vi "IviChannelsToProperty.vi"(8 "error in (no error)":errorcluster, 11 "IVI_Class.lvclass":refnum<class "IVI_Class.lvclass">) -> (0 "error out":errorcluster, 3 "IVI_Class.lvclass":refnum<class "IVI_Class.lvclass">)   [LabVIEW 2014, in "ScopePlugins.lvlib" / "IVI_Class.lvclass"]
doc: "Reads IVI Scope Acquisition properties and writes them into the Scope class Acquisition Properties"
uses:
  IVI_Class.lvclass
  ScopePluginBaseClass/ScopePluginsBase.lvclass/ScopePluginsBase.ctl
  ScopePluginBaseClass/Accessors/Write Channels.vi
  ScopePluginBaseClass/Accessors/Read Handle.vi
  ScopePluginBaseClass/Accessors/Read Connected.vi
  ScopePluginBaseClass/Accessors/Read Channels.vi
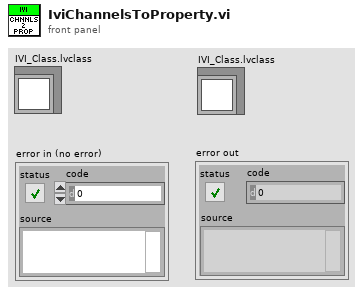
[diagram p1: front panel]
types:
  T1 = typedef "ScopePlugins.lvlib/Channels.ctl" = cluster{"Count":i32, "ChannelArray":T2[]}
  T2 = typedef "ScopePlugins.lvlib/Channel.ctl" = cluster{"Enabled":bool, "Name":string, "InputImpedance":dbl, "InputFreqMax":dbl, "ProbeAttn":dbl, "Coupling":enum16{"AC", "DC", "GND"}, "Offset":dbl, "Range":dbl}
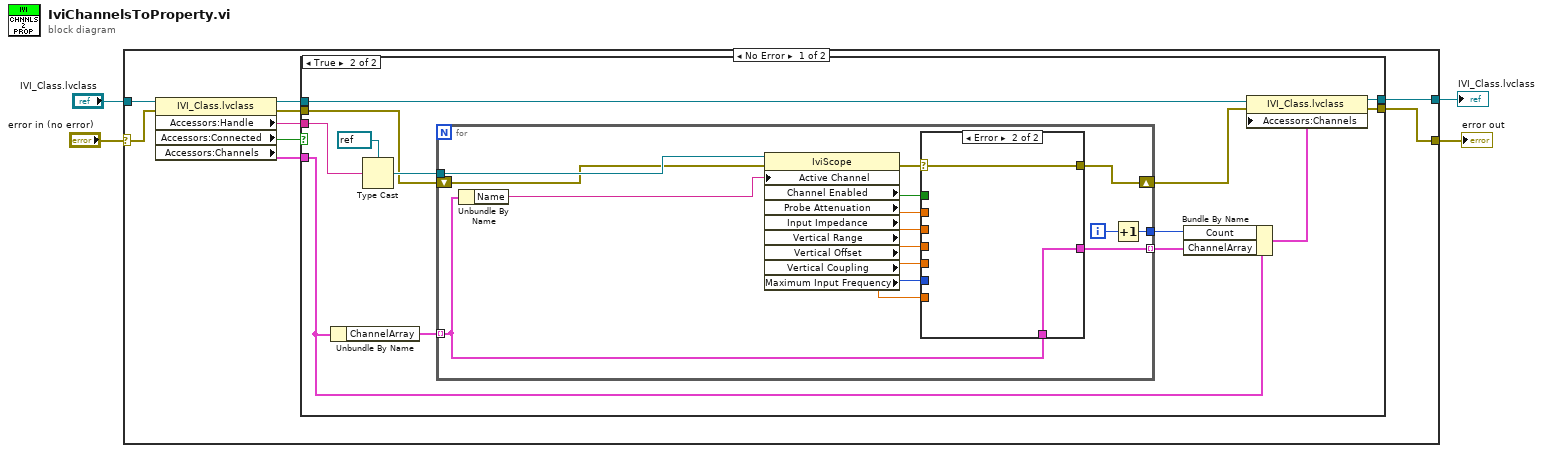
[diagram p0: block diagram]
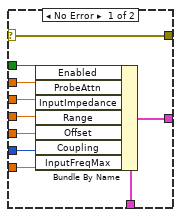
[diagram p3: hidden frame]
diagram:
  n1 = case shown="No Error" "error in (no error)" {
    selector: "error in (no error)" -> [w9 w57]
    tunnel: "IVI_Class.lvclass" -> [w13 w58]
    tunnel: [w10 w58] -> w3
    tunnel: [w7 w57] -> w1
    frame No Error {
      n2 = property class="IVI_Class.lvclass"(reference=w13, error in=w9) -> (reference out=w11:refnum<class "IVI_Class.lvclass">, error out=w8:errorcluster, "Accessors:Handle"=w12:string, "Accessors:Connected"=w6:bool, "Accessors:Channels"=w5:T1)
      n3 = case shown="True" w6 {
        tunnel: w12 -> [_ w27]
        tunnel: w11 -> [w15 w20]
        tunnel: [w15 w25] -> w10
        tunnel: w8 -> [w14 w24]
        tunnel: [w14 w22] -> w7
        tunnel: w5 -> [_ w19]
        frame False {
        }
        frame True {
          n4 = Unbundle By Name(w19) -> ("ChannelArray"=w21:T2[])
          n5 = Type Cast(type=refnum<k15> refnum ("reference out"), x=w27) -> (*(type *) &x=w26:refnum<k15>)
          n6 = for {
            tunnel: w26 -> [w39]
            shift-right: [w40] -> w23
            shift-left: w24 -> [w38]
            tunnel: w21 -> [w44] mode=indexing
            tunnel: [w43] -> w18 mode=indexing
            tunnel: [w29] -> w16
            i -> [w42]
            n7 = Unbundle By Name(w44) -> ("Name"=w37:string)
            n8 = property class="IviScope"(reference=w39, error in=w38, "Active Channel"=w37) -> (error out=w41:errorcluster, "Channel Enabled"=w36:bool, "Probe Attenuation"=w35:dbl, "Input Impedance"=w34:dbl, "Vertical Range"=w33:dbl, "Vertical Offset"=w32:dbl, "Vertical Coupling"=w31:i32, "Maximum Input Frequency"=w30:dbl)  [unwired: 1 out]
            n9 = case shown="Error" w41 {
              selector: w41 -> [w46 w56]
              tunnel: w44 -> [w54 w55]
              tunnel: [w53 w55] -> w43
              tunnel: w35 -> [w52 _]
              tunnel: w33 -> [w51 _]
              tunnel: w32 -> [w50 _]
              tunnel: w31 -> [w49 _]
              tunnel: w30 -> [w48 _]
              tunnel: w34 -> [w47 _]
              tunnel: [w46 w56] -> w40
              tunnel: w36 -> [w45 _]
              frame No Error {
                n10 = Bundle By Name(cluster=w54, "Enabled"=w45, "ProbeAttn"=w52, "InputImpedance"=w47, "Range"=w51, "Offset"=w50, "Coupling"=w49, "InputFreqMax"=w48) -> (w53:T2)
              }
              frame Error {
              }
            }
            n11 = Increment(x=w42) -> (x+1=w29:i32)
          }
          n12 = Bundle By Name(cluster=w19, "Count"=w16, "ChannelArray"=w18) -> (w17:T1)
          n13 = property class="IVI_Class.lvclass"(reference=w20, error in=w23, "Accessors:Channels"=w17) -> (reference out=w25:refnum<class "IVI_Class.lvclass">, error out=w22:errorcluster)
        }
      }
    }
    frame Error {
    }
  }
  "IVI_Class.lvclass" <- w3
  "error out" <- w1
